vi "Scale (SubVI).vi"(1 "Desired Angle":i16) -> (0 "Servo Out":u16)   [LabVIEW 2015]
doc: "Scaling UI from 0-180 into 0-1"
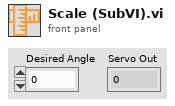
[diagram p1: front panel]
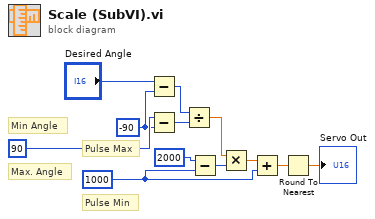
[diagram p0: block diagram]
diagram:
  w3 = 1000
  w10 = -90
  # "Pulse Max"
  # "Pulse Min"
  # "Max. Angle"
  # "Min Angle"
  n1 = Subtract(x="Desired Angle", y=w10) -> (x-y=w9:i32)
  n2 = Subtract(x=90, y=w10) -> (x-y=w8:i32)
  n3 = Divide(x=w9, y=w8) -> (x/y=w6:dbl)
  n4 = Subtract(x=2000, y=w3) -> (x-y=w5:i32)
  n5 = Multiply(x=w6, y=w5) -> (x*y=w4:dbl)
  n6 = Add(x=w4, y=w3) -> (x+y=w2:dbl)
  n7 = Round To Nearest(number=w2) -> (nearest integer value=→"Servo Out":dbl)
